vi "OTA WirelessServo Example 2.vi"() -> ()   [LabVIEW 2014]
uses:
  LabVIEW-Universal-Transcriptor-ServoLibrary/ServoDatatype.lvclass
  <vilib>/LabVIEW Universal Transcriptor/LabVIEW to Arduino Transcriptor/Transcriptors/System API/Serial println string.vi
  <vilib>/LabVIEW Universal Transcriptor/ESP8266 WiFi Wrapper/ESP8266 WiFi Wrapper.lvlib
panel:
  out "Error Out":errorcluster
  out "Numeric":i8
  in  "DNS address":u8[](array[numeric])=[1, 2, 3, 4]
  in  "IP address":u8[](array[numeric])=[192, 168, 0, 42]
  in  "Gateway":u8[](array[numeric])=[192, 168, 0, 1]
  in  "Subnet mask":u8[](array[numeric])=[255, 255, 255, 0]
  in  "Password":string="12345678"
  in  "SSID":string="ESP8266 Wifi Example"
  in  "Listen Port":u8=80
  in  "error in (no error)":errorcluster
  # "This example creates server and listen to command.\nRotate servo is: IPADDR/servoXXX\n    - where XXX are three ciphers which are angle\n    - IPADDR/servo000 = rotate to 0deg\n    - IPADDR/servo090 = rotate to 90deg\n    - IPADDR/servo180 = rotate to 180deg"
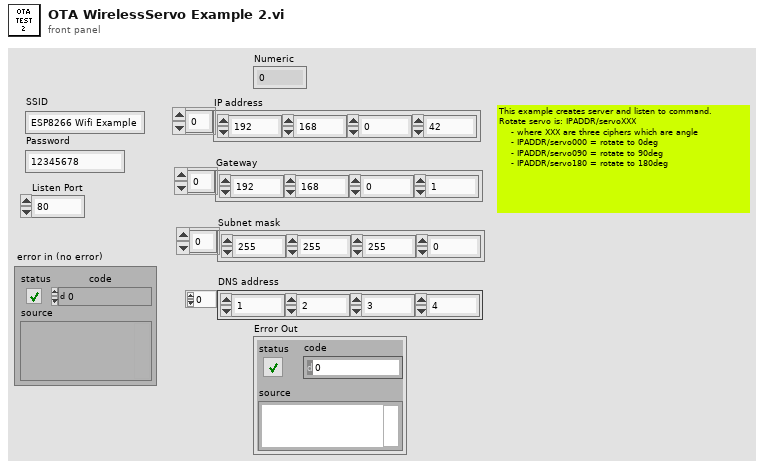
[diagram p1: front panel]
types:
  T1 = enum16{"WIFI_OFF", "WIFI_STA", "WIFI_AP", "WIFI_AP_STA"}
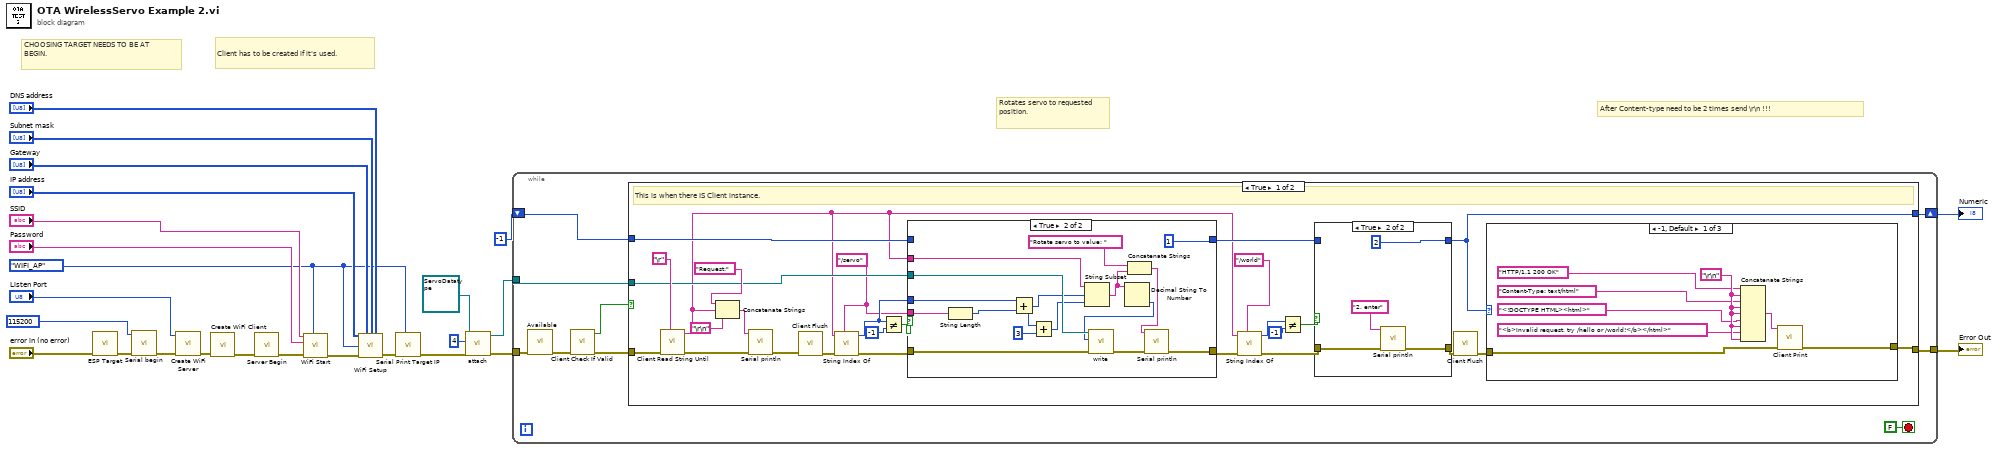
[diagram p0: block diagram]
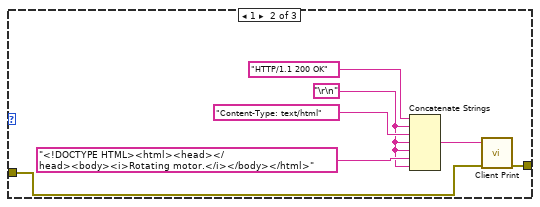
[diagram p2: hidden frame]
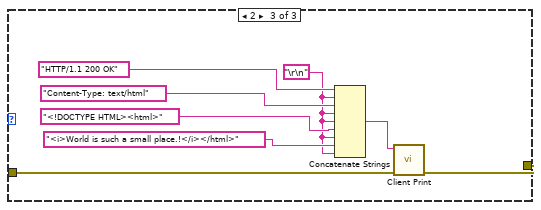
[diagram p3: hidden frame]
diagram:
  w12 = T1."WIFI_AP" ("WiFi Server Mode")
  # "After Content-type need to be 2 times send \\r\\n !!!"
  # "Rotates servo to requested position."
  # "CHOOSING TARGET NEEDS TO BE AT BEGIN."
  # "Client has to be created if it's used."
  n1 = call <vilib>:"ESP Target.vi"("Error In"="error in (no error)") -> ("Error Out"=w10:errorcluster)  [unwired: 10 in]
  n2 = call <vilib>:"Serial begin.vi"("Error In"=w10, "speed (Bd)"=115200 ("Speed")) -> ("Error Out"=w11:errorcluster)  [unwired: 9 in]
  n3 = call <vilib>:"Create WiFi Server.vi"("Error In"=w11, "Listen Port"="Listen Port") -> ("Error Out"=w23:errorcluster)  [unwired: 9 in]
  n4 = call <vilib>:"Create WiFi Client.vi"("Error In"=w23) -> ("Error Out"=w19:errorcluster)  [unwired: 10 in]
  n5 = call <vilib>:"Server Begin.vi"("Error In"=w19) -> ("Error Out"=w21:errorcluster)  [unwired: 10 in]
  n6 = call <vilib>:"WiFi Start.vi"("WiFi Mode"=w12, "Error In"=w21, "Password"="Password", "SSID"="SSID") -> ("Error Out"=w20:errorcluster)  [unwired: 7 in]
  n7 = call <vilib>:"WiFi Setup.vi"("IP address"="IP address", "Gateway address"="Gateway", "Subnet mask"="Subnet mask", "DNS address"="DNS address", "WiFi Mode"=w12, "Error In"=w20) -> ("Error Out"=w5:errorcluster)  [unwired: 9 in]
  n8 = call <vilib>:"Serial Print Target IP.vi"("WiFi Mode"=w12, "Error In"=w5) -> ("Error Out"=w6:errorcluster)  [unwired: 9 in]
  n9 = call-dynamic "attach.vi"("error in (no error)"=w6, "pin number"=4, "Servo in"=refnum<class "ServoDatatype.lvclass"> refnum) -> ("error out"=w2:errorcluster, "Servo out"=w1:refnum<class "ServoDatatype.lvclass">)  [unwired: 6 in, 1 out]
  n10 = while {
    tunnel: [w32] -> w7
    shift-right: [w30] -> w8
    shift-left: i8 -1 -> [w31]
    tunnel: w2 -> [w28]
    tunnel: w1 -> [w26]
    stop <- FALSE stop-if-true
    n11 = call <vilib>:"Available.vi"("Error In"=w28) -> ("Error Out"=w27:errorcluster)  [unwired: 10 in]
    n12 = call <vilib>:"Client Check If Valid.vi"("Error In"=w27) -> ("Error Out"=w29:errorcluster, "Is Null?"=w33:bool)  [unwired: 9 in]
    n13 = case shown="True" w33 {
      tunnel: w29 -> [w61 w110]
      tunnel: [w42 w110] -> w32
      tunnel: [w46 w109] -> w30
      tunnel: w31 -> [w49 w109]
      tunnel: w26 -> [w38 _]
      frame True {
        w35 = "/servo" ("IndexOf String")
        # "This is when there IS Client instance."
        n14 = call <vilib>:"Client Read String Until.vi"("Terminator char"="\r" ("Carriage Return Constant"), "Error In"=w61) -> ("Error Out"=w40:errorcluster, "Read String"=w37:string)  [unwired: 8 in]
        n15 = Concatenate Strings("Request:" ("string"), w37, "\r\n" ("End of Line Constant")) -> (w39:string)
        n16 = call-poly <vilib>:"Serial println.vi"("Error In"=w40, "string in"=w39) -> ("Error Out"=w41:errorcluster)  [unwired: 9 in]
        n17 = call <vilib>:"Client Flush.vi"("Error In"=w41) -> ("Error Out"=w59:errorcluster)  [unwired: 10 in]
        n18 = call <vilib>:"String Index Of.vi"("IndexOf String"=w35, "Error In"=w59, "Input String"=w37) -> ("Error Out"=w56:errorcluster, "index"=w36:i8)  [unwired: 7 in]
        n19 = Not Equal?(x=w36, y=i8 -1) -> (x != y?=w58:bool)
        n20 = case shown="True" w58 {
          tunnel: [w92 w107] -> w50
          tunnel: w56 -> [w92 w105]
          tunnel: [w91 i8 1] -> w48
          tunnel: w49 -> [w91 _]
          tunnel: w38 -> [_ w104]
          tunnel: w37 -> [_ w103]
          tunnel: w36 -> [_ w98]
          tunnel: w35 -> [_ w94]
          frame False {
          }
          frame True {
            n21 = String Length(string=w94) -> (length=w95:i32)
            n22 = Add(x=w98, y=w95) -> (x+y=w97:i32)
            n23 = Add(x=w97, y=i8 3) -> (x+y=w93:i32)
            n24 = String Subset(string=w103, offset (0)=w97, length (rest)=w93) -> (substring=w101:string)
            n25 = Decimal String To Number(string=w101) -> (number=w102:i32)  [unwired: 2 in, 1 out]
            n26 = call-dynamic "write.vi"("error in (no error)"=w105, "value"=w102, "ServoDatatype in"=w104) -> ("error out"=w106:errorcluster)  [unwired: 7 in, 1 out]
            n27 = Concatenate Strings("Rotate servo to value: " ("string"), w101) -> (w100:string)
            n28 = call-poly <vilib>:"Serial println.vi"("Error In"=w106, "string in"=w100) -> ("Error Out"=w107:errorcluster)  [unwired: 9 in]
          }
        }
        n29 = call <vilib>:"String Index Of.vi"("IndexOf String"="/world", "Error In"=w50, "Input String"=w37) -> ("Error Out"=w55:errorcluster, "index"=w52:i8)  [unwired: 7 in]
        n30 = Not Equal?(x=w52, y=i8 -1) -> (x != y?=w53:bool)
        n31 = case shown="True" w53 {
          tunnel: [w86 w88] -> w47
          tunnel: w55 -> [w86 w87]
          tunnel: [w85 i8 2] -> w46
          tunnel: w48 -> [w85 _]
          frame False {
          }
          frame True {
            n32 = call-poly <vilib>:"Serial println.vi"("Error In"=w87, "string in"="2. enter" ("String")) -> ("Error Out"=w88:errorcluster)  [unwired: 9 in]
          }
        }
        n33 = call <vilib>:"Client Flush.vi"("Error In"=w47) -> ("Error Out"=w45:errorcluster)  [unwired: 10 in]
        n34 = case shown="-1, Default" w46 {
          tunnel: [w68 w76 w83] -> w42
          tunnel: w45 -> [w69 w72 w84]
          frame -1, Default {
            w67 = "\r\n" ("End of Line Constant")
            # "After Content-type need to be 2 times send \\r\\n !!!"
            n35 = Concatenate Strings("HTTP/1.1 200 OK", w67, "Content-Type: text/html", w67, w67, "<!DOCTYPE HTML><html>", w67, "<b>Invalid request, try /hello or /world!</b></html>", w67) -> (w62:string)
            n36 = call <vilib>:"Client Print.vi"("Error In"=w69, "Input String"=w62) -> ("Error Out"=w68:errorcluster)  [unwired: 9 in]
          }
          frame 1 {
            w70 = "\r\n" ("End of Line Constant")
            n37 = Concatenate Strings("HTTP/1.1 200 OK", w70, "Content-Type: text/html", w70, w70, "<!DOCTYPE HTML><html><head></head><body><i>Rotating motor.</i></body></html>", w70) -> (w71:string)
            n38 = call <vilib>:"Client Print.vi"("Error In"=w72, "Input String"=w71) -> ("Error Out"=w76:errorcluster)  [unwired: 9 in]
          }
          frame 2 {
            w78 = "\r\n" ("End of Line Constant")
            n39 = Concatenate Strings("HTTP/1.1 200 OK", w78, "Content-Type: text/html", w78, w78, "<!DOCTYPE HTML><html>", w78, "<i>World is such a small place.!</i></html>", w78) -> (w77:string)
            n40 = call <vilib>:"Client Print.vi"("Error In"=w84, "Input String"=w77) -> ("Error Out"=w83:errorcluster)  [unwired: 9 in]
          }
        }
      }
      frame False {
        # "No Client instance, do nothing."
      }
    }
  }
  "Numeric" <- w8
  "Error Out" <- w7
